vi "Delete Logged Files.vi"() -> ()   [LabVIEW 2020]
uses:
  <vilib>/Skyline/File/HTTP/NI Skyline File HTTP.lvclass
  C:/Program Files (x86)/National Instruments/LabVIEW 2020/vi.lib/Skyline/File/Base/NI Skyline File Base.lvclass
  <vilib>/Skyline/File/Filter/Create Filter (Name).vi
  <vilib>/Skyline/File/Filter/Create Filter (Extension).vi
  <vilib>/Skyline/File/File/Delete (Multiple).vi
  <vilib>/Skyline/File/File/NI Skyline File.lvclass
  <vilib>/Skyline/File/Filter/NI Skyline File Filter.lvclass
  C:/Program Files (x86)/National Instruments/LabVIEW 2020/vi.lib/Skyline/File/HTTP/NI Skyline File HTTP.lvclass
panel:
  out "Numeric":i32
  out "size(s)":i32
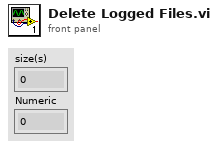
[diagram p1: front panel]
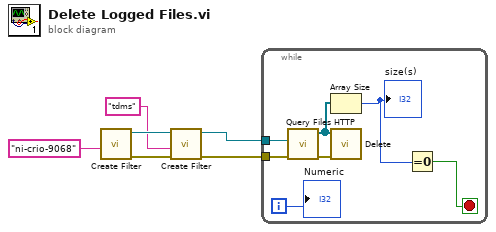
[diagram p0: block diagram]
diagram:
  n1 = call-poly <vilib>:"Create Filter.vi"("value"="ni-crio-9068") -> ("error out"=w5:errorcluster, "filter out"=w2:refnum<class "NI Skyline File Filter.lvclass">)  [unwired: 9 in]
  n2 = call-poly <vilib>:"Create Filter.vi"("error in (no error)"=w5, "value"="tdms", "filter in"=w2) -> ("error out"=w4:errorcluster, "filter out"=w3:refnum<class "NI Skyline File Filter.lvclass">)  [unwired: 7 in]
  n3 = while {
    tunnel: w4 -> [w11]
    tunnel: w3 -> [w10]
    i -> [w7]
    stop <- w8 stop-if-true
    n4 = call <vilib>:"Query Files HTTP.vi"("error in (no error)"=w11, "filter in"=w10) -> ("error out"=w12:errorcluster, "files"=w13:refnum<class "NI Skyline File HTTP.lvclass">[])  [unwired: 7 in, 1 out]
    n5 = Array Size(array=w13) -> (size(s)=w9:i32)
    "size(s)" <- w9
    n6 = call-poly <vilib>:"Delete.vi"("error in (no error)"=w12, "files"=w13) -> ()  [unwired: 9 in, 1 out]
    n7 = Equal To 0?(x=w9) -> (x = 0?=w8:bool)
    "Numeric" <- w7
  }
